vi "Intellifaucet_Control.vi"(7 "Type":T1, 8 "error in (no error)":errorcluster, 11 "Queue in":refnum<queue>) -> (0 "error out":errorcluster, 3 "Queue out":refnum<queue>)   [LabVIEW 2020]
uses:
  Message Queue/Message Cluster.ctl
  StartStopIntellifaucet.ctl
  Message Queue/Enqueue Message (Single).vi
  Message Queue/Message Queue.lvlib
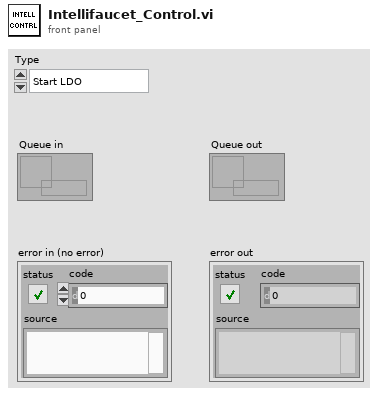
[diagram p1: front panel]
types:
  T1 = typedef "StartStopIntellifaucet.ctl" = enum16{"Start LDO", "Stop LDO", "Start FVIR", "Stop FVIR"}
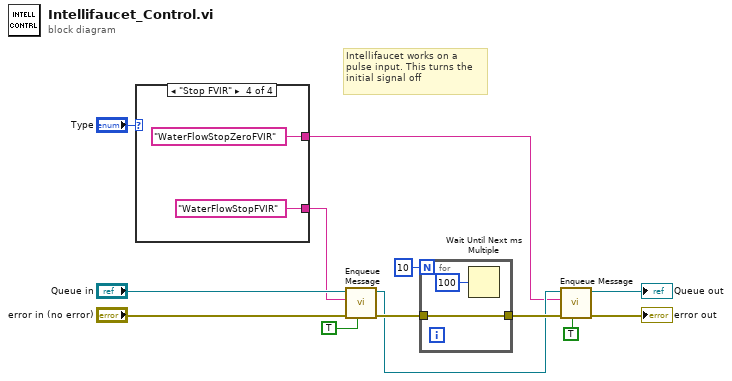
[diagram p0: block diagram]
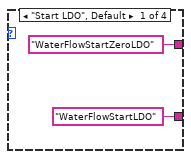
[diagram p2: hidden frame]
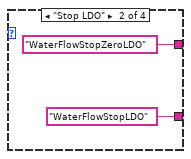
[diagram p3: hidden frame]
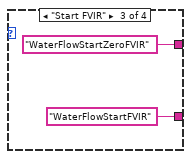
[diagram p4: hidden frame]
diagram:
  # "Intellifaucet works on a\npulse input. This turns the \ninitial signal off"
  n1 = case shown="\"Stop FVIR\"" "Type" {
    tunnel: ["WaterFlowStartLDO" ("Message") "WaterFlowStopLDO" ("Message") "WaterFlowStartFVIR" ("Message") "WaterFlowStopFVIR" ("Message")] -> w4
    tunnel: ["WaterFlowStartZeroLDO" ("Message") "WaterFlowStopZeroLDO" ("Message") "WaterFlowStartZeroFVIR" ("Message") "WaterFlowStopZeroFVIR" ("Message")] -> w3
    frame "Start LDO", Default {
    }
    frame "Stop LDO" {
    }
    frame "Start FVIR" {
    }
    frame "Stop FVIR" {
    }
  }
  n2 = call-poly "Enqueue Message.vi"("Priority Message? (F)"=TRUE, "error in (no error)"="error in (no error)", "Message"=w4, "Message Queue"="Queue in") -> ("error out"=w11:errorcluster, "dup Message Queue"=w7:refnum<queue>)  [unwired: 6 in]
  n3 = for {
    N: 10 -> [_]
    tunnel: w11 -> [w22]
    tunnel: [w22] -> w12
    n4 = Wait Until Next ms Multiple(millisecond multiple=u32 100) -> ()  [unwired: 1 out]
  }
  n5 = call-poly "Enqueue Message.vi"("Priority Message? (F)"=TRUE, "error in (no error)"=w12, "Message"=w3, "Message Queue"=w7) -> ("error out"=→"error out":errorcluster, "dup Message Queue"=→"Queue out":refnum<queue>)  [unwired: 6 in]
